vi "Configure Current Trigger Level.vi"(8 "error in":errorcluster, 9 "Level(A)":dbl min=0.0 format="%.2g", 11 "VISA resource name":refnum<visa-resource-name>) -> (0 "error out":errorcluster, 3 "VISA resource name out":refnum<visa-resource-name>)   [LabVIEW 2015, in "IT6700H.lvlib"]
doc: "This command is used to set a current value waiting to be triggered. This value is stored until a trigger signal is received and the power supply outputs at this current value. Sending the CURRent command does not affect the value set by this command. When the query command is sent, the value set before is returned. If the value is not set before, the value set by the CURRent command is returned. Send CURR:TRIG? MAX or CURR:TRIG? MIN returns the maximum or minimum current value that can be set.\n<b>Level(A)</b>\n0-MAX"
uses:
  <instrlib>/IT6700H/IT6700H.lvlib
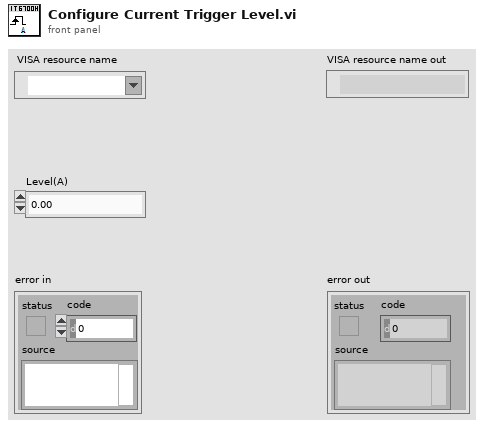
[diagram p1: front panel]
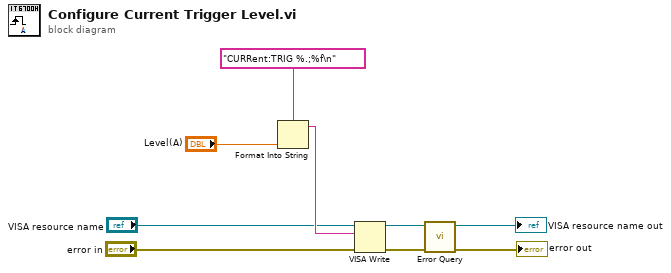
[diagram p0: block diagram]
diagram:
  n1 = Format Into String(format string="CURRent:TRIG %.;%f\n", "Level(A)") -> (resulting string=w7:string)  [unwired: 2 in, 1 out]
  n2 = VISA Write(VISA resource name="VISA resource name", write buffer=w7, error in (no error)="error in") -> (VISA resource name out=w3:refnum<visa-resource-name>, error out=w4:errorcluster)  [unwired: 1 out]
  n3 = call <instrlib>:"Error Query.vi"("error in"=w4, "VISA resource name"=w3) -> ("error out"=→"error out":errorcluster, "VISA resource name out"=→"VISA resource name out":refnum<visa-resource-name>)  [unwired: 6 in, 2 out]
